vi "Relay Control.vi"(0 "VISA resource name":refnum<visa-resource-name>, 5 "Relay Contacts(F:Close)":bool, 11 "error in (no error)":errorcluster, 12 "Polarity(F:Normal)":bool) -> (4 "VISA resource name out":refnum<visa-resource-name>, 15 "error out":errorcluster)   [LabVIEW 2012, in "Agilent 66XX Series.lvlib"]
doc: "These commands control the optional HP Relay Accessories. If the power supply is not configured for the optional relay connector, an error will occur and can be found using the error query vi. CAUTION: For models 664x,665x,667x,668x.669x do not install or use this VI if the power supply maximum output current rating exceeds the contact ratings of the relays."
uses:
  <instrlib>/Agilent 66XX Series/Agilent 66XX Series.lvlib
panel:
  # "Open"
  # "Close"
  # "Reverse"
  # "Normal"
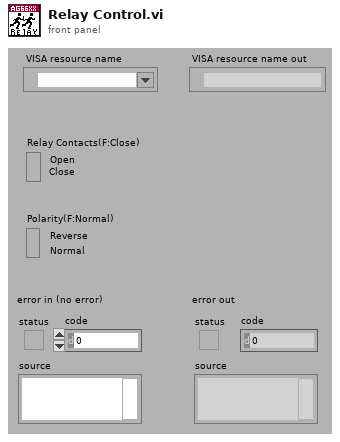
[diagram p1: front panel]
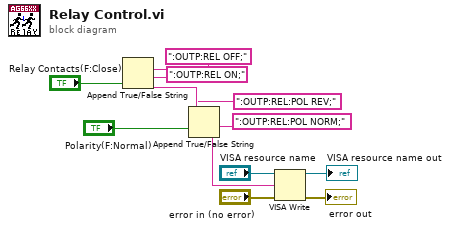
[diagram p0: block diagram]
diagram:
  n1 = Append True/False String(1:"Relay Contacts(F:Close)", 2:":OUTP:REL ON;", 3:":OUTP:REL OFF;") -> (0:w9:string)  [unwired: 1 in]
  n2 = Append True/False String(1:"Polarity(F:Normal)", 2:":OUTP:REL:POL NORM;", 3:":OUTP:REL:POL REV;", 4:w9) -> (0:w3:string)
  n3 = VISA Write(VISA resource name="VISA resource name", write buffer=w3, error in (no error)="error in (no error)") -> (VISA resource name out=→"VISA resource name out":refnum<visa-resource-name>, error out=→"error out":errorcluster)  [unwired: 1 out]
